vi "Generate AsyncMsg Event_DAQ.vi"(8 "error in (no error)":errorcluster, 9 "vData":variant, 10 "AsyncMsg":T1, 11 "DAQ":refnum<class "DAQ.lvclass">) -> (0 "error out":errorcluster, 3 "DAQ out":refnum<class "DAQ.lvclass">)   [LabVIEW 2022 SP3, in "DAQ.lvclass"]
doc: "Developed by Kevin Thompson\nkevin@thompsonengineering.net\n\nCopyright 2018-2020\nThompson Engineering, LLC"
uses:
  DAQ.lvclass
  DataTypes/AsyncMsg_DAQ--enum.ctl
  Common/Controls/TD Async CmdMsg EventData--cluster.ctl
  DAQ.lvclass/DAQ.ctl
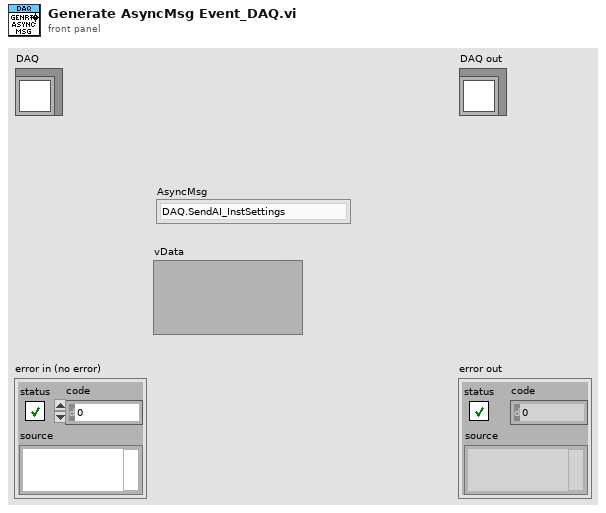
[diagram p1: front panel]
types:
  T1 = typedef "DAQ.lvclass/AsyncMsg_DAQ--enum.ctl" = enum16{"DAQ.SendAI_InstSettings"}
  T2 = typedef "TD Async CmdMsg EventData--cluster.ctl" = cluster{"Time Stamp":timestamp, "CmdMsg":string, "vData":variant}
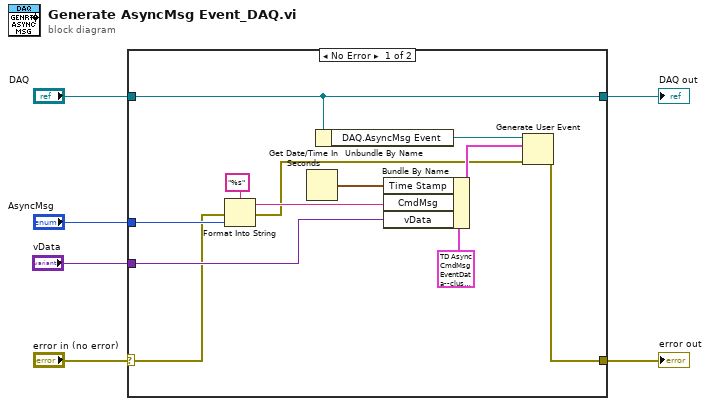
[diagram p0: block diagram]
diagram:
  n1 = case shown="No Error" "error in (no error)" {
    selector: "error in (no error)" -> [w8 w20]
    tunnel: [w17 w20] -> w5
    tunnel: [w9 w19] -> w3
    tunnel: "DAQ" -> [w9 w19]
    tunnel: "AsyncMsg" -> [w12 _]
    tunnel: "vData" -> [w10 _]
    frame No Error {
      n2 = Format Into String(format string="%s", error in=w8, w12) -> (resulting string=w11:string, error out=w7:errorcluster)  [unwired: 1 in]
      n3 = Get Date/Time In Seconds() -> (seconds since 1Jan1904=w14:timestamp)
      n4 = Unbundle By Name(w9) -> ("DAQ.AsyncMsg Event"=w18:refnum<user-event>)
      n5 = Bundle By Name(cluster=T2 {"Time Stamp"=timestamp(0 s since 1904-01-01), "CmdMsg"="", "vData"=variant} ("Async EvData"), "Time Stamp"=w14, "CmdMsg"=w11, "vData"=w10) -> (w16:T2)
      n6 = Generate User Event(user event=w18, event data cluster=w16, error in=w7) -> (error out=w17:errorcluster)  [unwired: 1 in, 1 out]
    }
    frame Error {
    }
  }
  "error out" <- w5
  "DAQ out" <- w3
